vi "BSAs to communicate with.vi"(3 "LDA Channels":T1[](array[typedef]) {"Sync Delay (s)" format="%.2g"; "Req Sampling Rate Hz" min=1.0; "Shifted mW" format="%.1g"; "Unshifted mW" format="%.1g"; "Centre Velocity (m/s)" format="%.2g"; "Velocity Range (m/s)" format="%.2g"; "Focal Length (mm)" format="%.1f"; "Beam Separation (mm)" format="%.1f"; "Optics Conversion Factor" format="%.3g"; "High voltage" min=0 max=2040 step=8; "Signal gain (dB)" min=0 max=30 step=1; "Min Velocity" format="%.2g"; "Max Velocity" format="%.2g"; "Wavelength (nm)" format="%.1f"}) -> (1 "BSAs to contact":cluster{T1[]}[](array[cluster]) {"?"."Sync Delay (s)" format="%.2g"; "?"."Req Sampling Rate Hz" min=1.0; "?"."Shifted mW" format="%.1g"; "?"."Unshifted mW" format="%.1g"; "?"."Centre Velocity (m/s)" format="%.2g"; "?"."Velocity Range (m/s)" format="%.2g"; "?"."Focal Length (mm)" format="%.1f"; "?"."Beam Separation (mm)" format="%.1f"; "?"."Optics Conversion Factor" format="%.3g"; "?"."High voltage" min=0 max=2040 step=8; "?"."Signal gain (dB)" min=0 max=30 step=1; "?"."Min Velocity" format="%.2g"; "?"."Max Velocity" format="%.2g"; "?"."Wavelength (nm)" format="%.1f"})   [LabVIEW 2022 SP3]
uses:
  LDA_Channel.ctl
  <vilib>/Utility/error.llb/Trim Whitespace One-Sided.vi
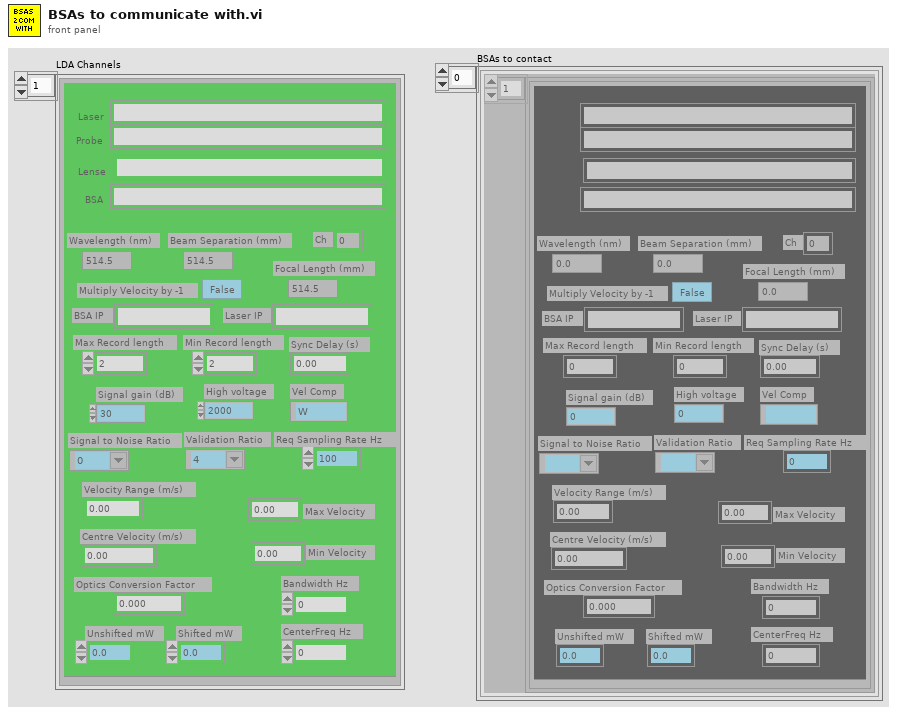
[diagram p1: front panel]
types:
  T1 = typedef "LDA_Channel.ctl" = cluster{"Wavelength (nm)":dbl, "Vel Comp":string, "Max Velocity":dbl, "Min Velocity":dbl, "Max Record length":u16, "Signal gain (dB)":i16, "High voltage":i16, "Optics Conversion Factor":dbl, "Min Record length":u16, "Multiply Velocity by -1":bool, "Signal to Noise Ratio":string, "Validation Ratio":string, "Probe":string, "Laser":string, "BSA":string, "Lense":string, "Beam Separation (mm)":dbl, "Focal Length (mm)":dbl, "COLOUR":u32, "BSA IP":string, "Velocity Range (m/s)":dbl, "Centre Velocity (m/s)":dbl, "Unshifted mW":dbl, "Shifted mW":dbl, "Bandwidth Hz":dbl, "Req Sampling Rate Hz":dbl, "Ch":i32, "CenterFreq Hz":dbl, "Laser IP":string, "Sync Delay (s)":dbl}
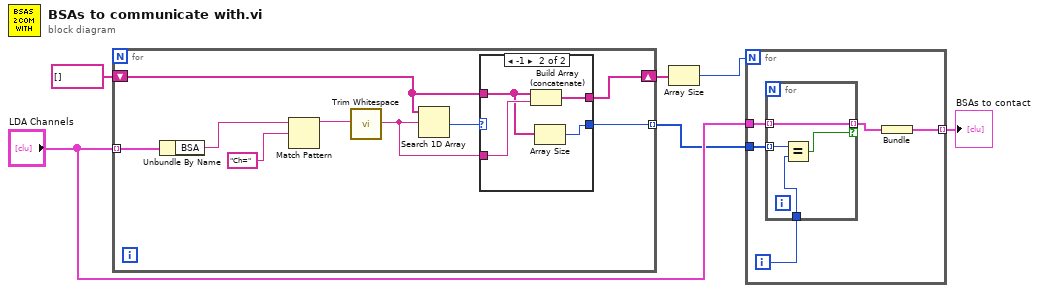
[diagram p0: block diagram]
diagram:
  n1 = for {
    tunnel: "LDA Channels" -> [w15] mode=indexing
    shift-right: [w9] -> w5
    shift-left: string[] [] -> [w11]
    tunnel: [w8] -> w2 mode=indexing
    n2 = Unbundle By Name(w15) -> ("BSA"=w14:string)
    n3 = Match Pattern(string=w14, regular expression="Ch=") -> (before substring=w10:string)  [unwired: 1 in, 3 out]
    n4 = call <vilib>:"Trim Whitespace.vi"("string"=w10) -> ("trimmed string"=w7:string)  [unwired: 1 in]
    n5 = Search 1D Array(1D array=w11, element=w7) -> (index of element=w12:i32)  [unwired: 1 in]
    n6 = case shown="-1" w12 {
      selector: w12 -> [w16 _]
      tunnel: w11 -> [w17 w19]
      tunnel: w7 -> [_ w21]
      tunnel: [w17 w20] -> w9
      tunnel: [w16 w18] -> w8
      frame Default {
      }
      frame -1 {
        n7 = Build Array (concatenate)(w19, w21) -> (w20:string[])
        n8 = Array Size(array=w19) -> (size(s)=w18:i32)
      }
    }
  }
  n9 = Array Size(array=w5) -> (size(s)=w4:i32)
  n10 = for {
    N: w4 -> [_]
    tunnel: "LDA Channels" -> [w26]
    tunnel: w2 -> [w24]
    tunnel: [w22] -> w1 mode=indexing
    i -> [w25]
    n11 = for {
      tunnel: w26 -> [w28] mode=indexing
      tunnel: w25 -> [w30]
      tunnel: w24 -> [w29] mode=indexing
      tunnel: [w28] -> w23 mode=indexing if=w27
      n12 = Equal?(x=w29, y=w30) -> (x = y?=w27:bool)
    }
    n13 = Bundle(w23) -> (w22:cluster{T1[]})  [unwired: 1 in]
  }
  "BSAs to contact" <- w1
